vi "AB_Close_VI_and_Library_Arrays.vi"(8 "error in":errorcluster, 10 "VIs":refnum<vi>[](array[refnum]), 11 "Libraries":refnum<vi>[](array[refnum])) -> (0 "error out":errorcluster)   [LabVIEW 2020]
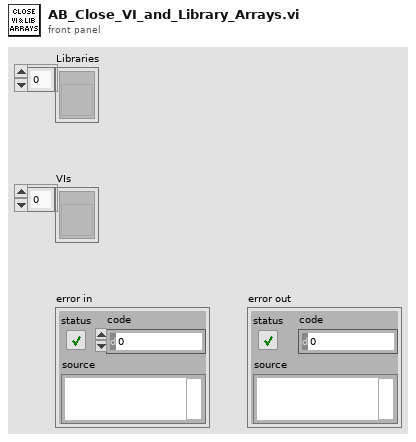
[diagram p1: front panel]
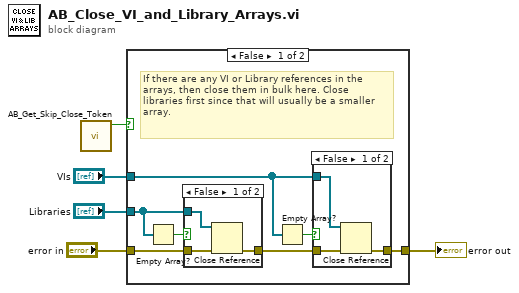
[diagram p0: block diagram]
diagram:
  n1 = call <vilib>:"AB_Get_Skip_Close_Token.vi"() -> ("Skip Close"=w3:bool)  [unwired: 10 in, 1 out]
  n2 = case shown="False" w3 {
    tunnel: [w11 w21] -> w5
    tunnel: "error in" -> [w12 w21]
    tunnel: "VIs" -> [w6 _]
    tunnel: "Libraries" -> [w8 _]
    frame False {
      # "If there are any VI or Library references in the arrays, then close them in bulk here. Close libraries first since that will usually be a smaller array."
      n3 = Empty Array?(array=w8) -> (empty?=w9:bool)
      n4 = case shown="False" w9 {
        tunnel: w12 -> [w19 w20]
        tunnel: [w18 w20] -> w10
        tunnel: w8 -> [w17 _]
        frame False {
          n5 = Close Reference(reference=w17, error in (no error)=w19) -> (error out=w18:errorcluster)
        }
        frame True {
        }
      }
      n6 = Empty Array?(array=w6) -> (empty?=w7:bool)
      n7 = case shown="False" w7 {
        tunnel: w10 -> [w15 w16]
        tunnel: [w14 w16] -> w11
        tunnel: w6 -> [w13 _]
        frame False {
          n8 = Close Reference(reference=w13, error in (no error)=w15) -> (error out=w14:errorcluster)
        }
        frame True {
        }
      }
    }
    frame True {
      # "INI token is present for skipping the Close Reference for VIs and Libraries."
    }
  }
  "error out" <- w5
